vi "MU Calibration Get Analog Master Track Adjustments.vi"(8 "error in (no error)":errorcluster, 11 "CalibrationHandle":T1) -> (0 "error out":errorcluster, 3 "masterAdjustments":T2)   [LabVIEW 2017, in "MU_3SL_interface.lvlib"]
doc: "MU_PUBLIC bool MU_Calibration_setCurrentAnalogTrackAdjustments(\n MU_Calibration* calibration,\n const MU_Calibration_AnalogTrackAdjustments* masterAdjustments,\n const MU_Calibration_AnalogTrackAdjustments* noniusAdjustments);"
uses:
  MU_3SL_interface.lvlib
  handles/CalibrationHandle.ctl
  lib/MU_3SL_interface.dll
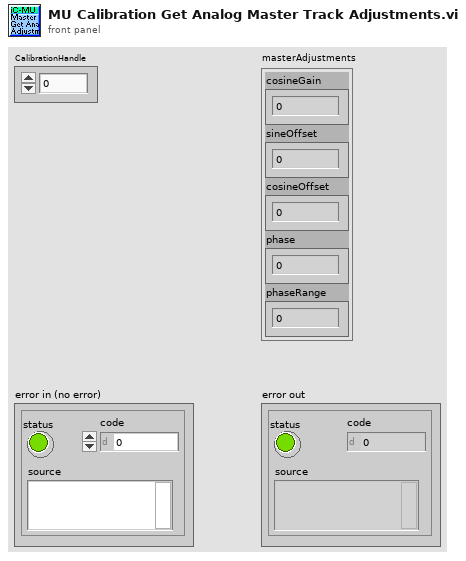
[diagram p1: front panel]
types:
  T1 = typedef "MU_3SL_interface.lvlib/CalibrationHandle.ctl" = u64
  T2 = cluster{"cosineGain":u8, "sineOffset":u8, "cosineOffset":u8, "phase":u8, "phaseRange":u8}
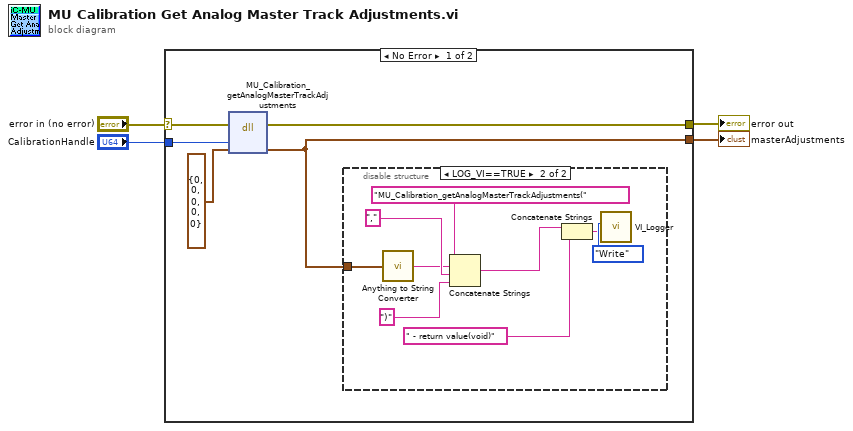
[diagram p0: block diagram]
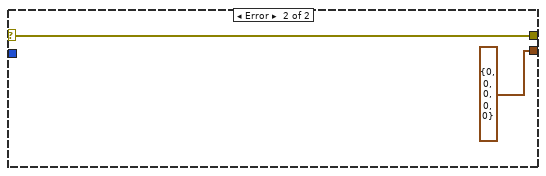
[diagram p3: hidden frame]
diagram:
  n1 = case shown="No Error" "error in (no error)" {
    selector: "error in (no error)" -> [w8 w20]
    tunnel: [w7 w20] -> w4
    tunnel: "CalibrationHandle" -> [w9 _]
    tunnel: [w5 T2 {"cosineGain"=0, "sineOffset"=0, "cosineOffset"=0, "phase"=0, "phaseRange"=0} ("masterAdjustments")] -> w1
    frame No Error {
      n2 = dll-call lib="C:/Users/bes/AppData/Roaming/work/mu_9so/icsubmodules/soft_mu_3sl_master/lv_interface/lib/MU_3SL_interface**.*" fn="MU_Calibration_getAnalogMasterTrackAdjustments"(error in=w8, "CalibrationHandle"=w9, "masterAdjustments"=T2 {"cosineGain"=0, "sineOffset"=0, "cosineOffset"=0, "phase"=0, "phaseRange"=0}) -> (error out=w7:errorcluster, "masterAdjustments"=w5:T2)  [unwired: 4 in, 1 out]
      n3 = disable-structure shown="LOG_VI==TRUE" {
        disable-tunnel: w5 -> [_ w13]
        frame condition #0 {
        }
        frame condition #1 (active) {
          n4 = call "Anything to String Converter.vi"("anything"=w13) -> ("String"=w12:string)
          n5 = Concatenate Strings("MU_Calibration_getAnalogMasterTrackAdjustments(" ("Info in"), w12, "," ("string"), ")" ("string")) -> (w11:string)
          n6 = Concatenate Strings(w11, " - return value(void)" ("string")) -> (w17:string)
          n7 = call "VI_Logger.vi"("Action (Read)"=enum16{"Write", "Read"}."Write", "Info in"=w17) -> ()  [unwired: 8 in, 2 out]
        }
      }
    }
    frame Error {
    }
  }
  "masterAdjustments" <- w1
  "error out" <- w4
